vi "Modefied Miller encoder.vi"(8 "Error In":errorcluster, 10 "Bit stream in":u8[](array[numeric])) -> (0 "error out":errorcluster {"code" format="Error %.0f"}, 2 "Bit stream out (NRZ encode)":u8[](array[numeric]))   [LabVIEW 2019]
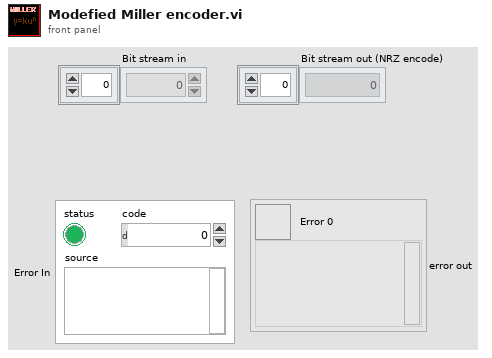
[diagram p1: front panel]
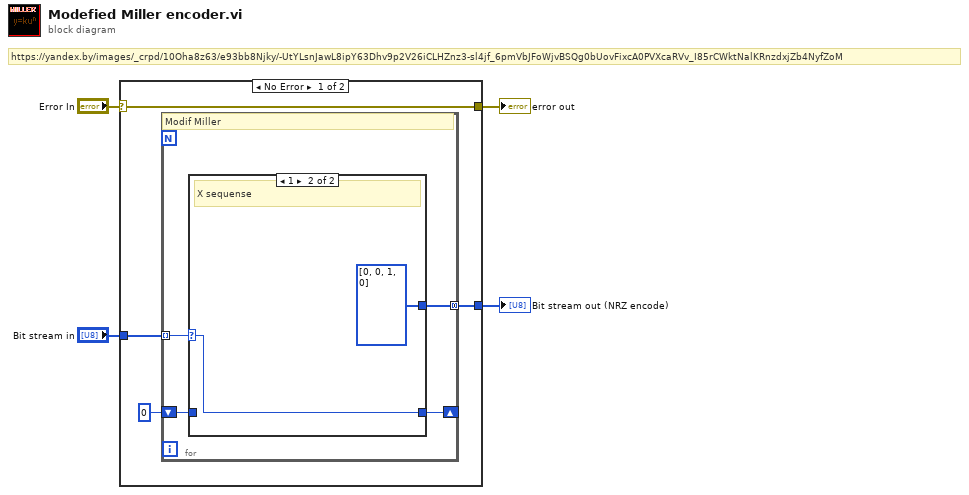
[diagram p0: block diagram]
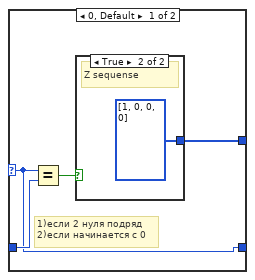
[diagram p2: hidden frame]
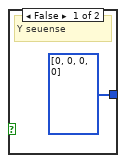
[diagram p3: hidden frame]
diagram:
  # "https://yandex.by/images/_crpd/10Oha8z63/e93bb8Njky/-UtYLsnJawL8ipY63Dhv9p2V26iCLHZnz3-sl4jf_6pmVbJFoWjvBSQg0bUovFixcA0PVXcaRVv_I85rCWktNalKRnzdxjZb4NyfZoM"
  n1 = case shown="No Error" "Error In" {
    selector: "Error In" -> [w8 w21]
    tunnel: "Bit stream in" -> [w6 _]
    tunnel: [w5 _] -> w3
    tunnel: [w8 w21] -> w1
    frame No Error {
      n2 = for {
        tunnel: w6 -> [w11] mode=indexing
        tunnel: [w12] -> w5 mode=concatenating
        shift-right: [w9] -> _
        shift-left: u8 0 -> [w10]
        # "Modif Miller"
        n3 = case shown="1" w11 {
          selector: w11 -> [w13 w19]
          tunnel: [w16 u8[] [0, 0, 1, 0] ("output array")] -> w12
          tunnel: w10 -> [w14 _]
          tunnel: [w13 w19] -> w9
          frame 0, Default {
            # "1)если 2 нуля подряд\n2)если начинается с 0"
            n4 = Equal?(x=w13, y=w14) -> (x = y?=w15:bool)
            n5 = case shown="True" w15 {
              tunnel: [u8[] [0, 0, 0, 0] ("output array") u8[] [1, 0, 0, 0] ("output array")] -> w16
              frame False {
                # "Y seuense"
              }
              frame True {
                # "Z sequense"
              }
            }
          }
          frame 1 {
            # "X sequense"
          }
        }
      }
    }
    frame Error {
    }
  }
  "Bit stream out (NRZ encode)" <- w3
  "error out" <- w1
